vi "Label Name.vi"(11 "Label Text":string) -> (3 "Variable Name":string)   [LabVIEW 2022 SP3, in "Interlocks.lvlib"]
uses:
  Interlocks.lvlib
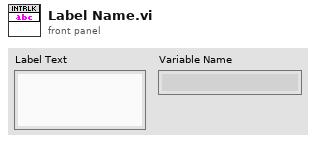
[diagram p1: front panel]
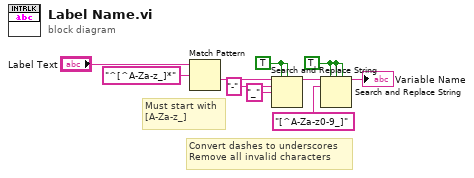
[diagram p0: block diagram]
diagram:
  w5 = TRUE ("replace all? (F)")
  w10 = TRUE ("replace all? (F)")
  # "Convert dashes to underscores\nRemove all invalid characters"
  # "Must start with\n[A-Za-z_]"
  n1 = Match Pattern(string="Label Text", regular expression="^[^A-Za-z_]*") -> (after substring=w1:string)  [unwired: 1 in, 3 out]
  n2 = Search and Replace String(replace all?=w5, case sensitive?=w5, input string=w1, search string="-", replace string="_" ("replace string (\"\")")) -> (result string=w7:string)  [unwired: 3 in, 3 out]
  n3 = Search and Replace String(replace all?=w10, case sensitive?=w10, multiline?=w10, input string=w7, search string="[^A-Za-z0-9_]") -> (result string=→"Variable Name":string)  [unwired: 3 in, 3 out]
